vi "ShooterTest.vi"(0 "Stop Button":bool, 7 "Shooter/ArmGripper (T/F)":bool, 9 "Shoot/Load":dbl(slide)=1500.0 scale=500.0..2500.0, 10 "pitch":dbl(slide)=850.0 scale=500.0..2500.0) -> (1 "Correct Key?":bool, 2 "Battery (Volts)":dbl format="%.1f")   [LabVIEW 2019]
uses:
  <vilib>/ReMiSYS/ReMiSYS_myRIO-mini/SubVI/SYS/servoPort.ctl
panel:
  out "error out":errorcluster
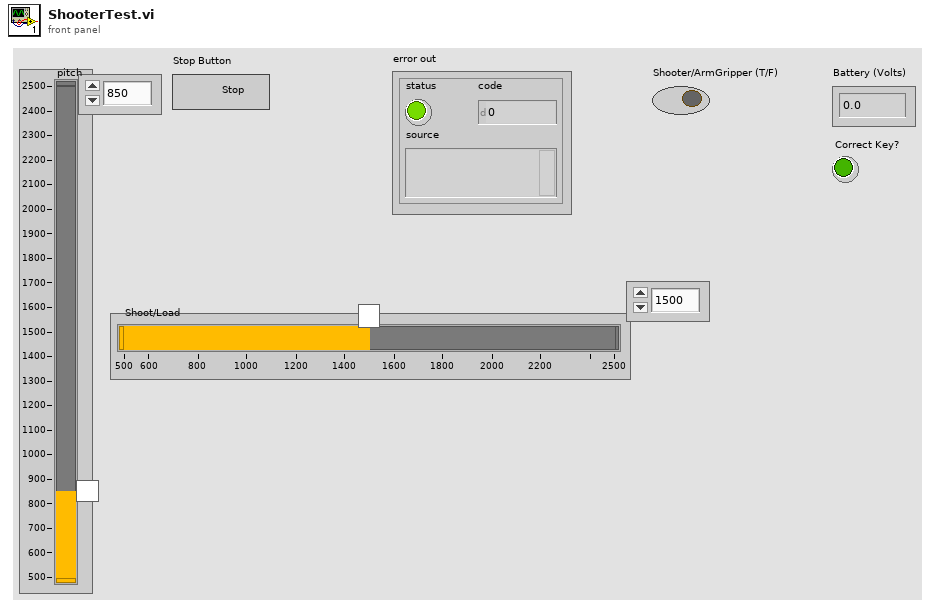
[diagram p1: front panel]
types:
  T1 = typedef "IMAQ Image.ctl" = refnum<image>
  T2 = typedef "IMAQ GM Match Report.ctl" = cluster{"Position":cluster{"x":sgl, "y":sgl}, "Angle":sgl, "Scale":sgl, "Score":sgl, "Bounding Box":cluster{"x":sgl, "y":sgl}[], "Contrast Reversed":bool, "Occlusion %":sgl, "Template Target Curve Score":sgl, "Target Template Curve Score":sgl, "Correlation Score":sgl}
  T3 = cluster{"Position":cluster{"x":sgl, "y":sgl}, "Angle":sgl, "Scale":sgl, "Score":sgl, "Bounding Box":cluster{"x":sgl, "y":sgl}[]}[]
  T4 = typedef "miniRef.ctl" = cluster{"Custom FPGA Reference":refnum<k20>, "error out":errorcluster}
  T5 = typedef "servoPort.ctl" = enum16{"S1", "S2", "S3", "S4", "S5", "S6", "S7", "S8", "S9"}
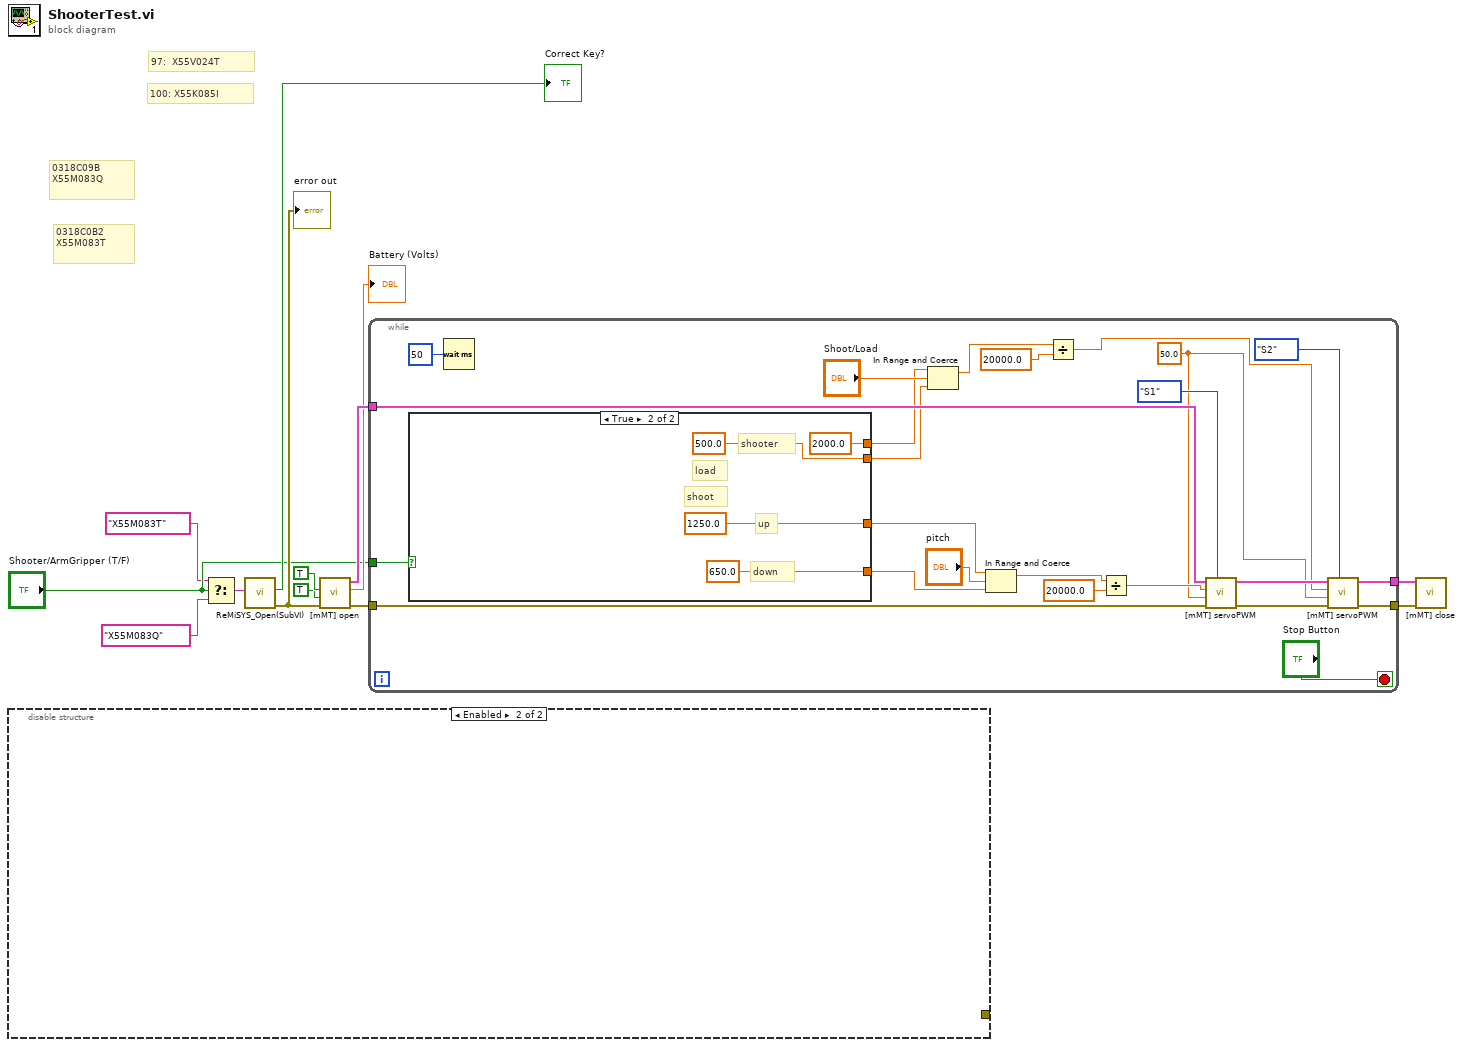
[diagram p0: block diagram]
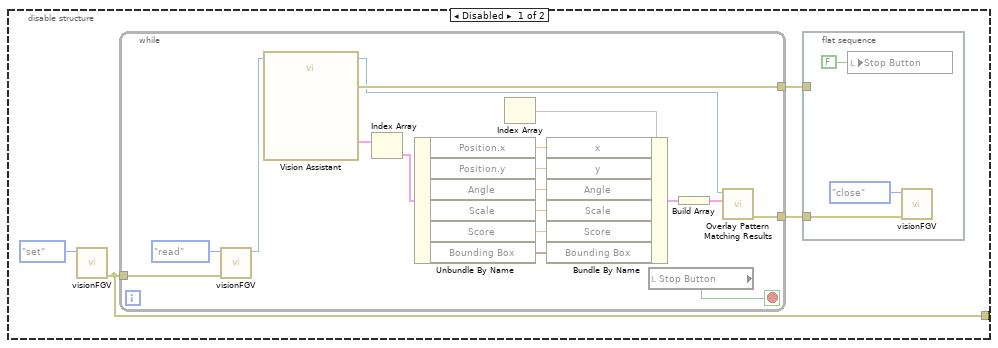
[diagram p2: hidden frame]
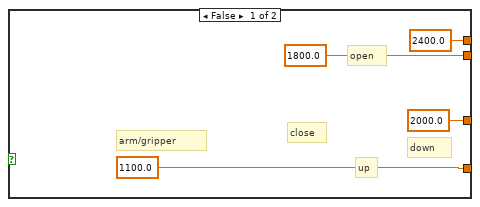
[diagram p3: hidden frame]
diagram:
  # "0318C0B2\nX55M083T"
  # "0318C09B\nX55M083Q"
  # "100: X55K085I"
  # "97:  X55V024T"
  n1 = disable-structure shown="Enabled" {
    disable-tunnel: [w16 _] -> _
    frame Disabled {
      n2 = call "visionFGV.vi"("Function"=enum16{"set", "read", "close"}."set") -> ("error out"=w16:errorcluster)  [unwired: 9 in, 1 out]
      n3 = while {
        tunnel: w16 -> [w38]
        tunnel: [w35] -> w15
        tunnel: [w21] -> w14
        stop <- w36 stop-if-true
        n4 = call "visionFGV.vi"("Error In"=w38, "Function"=enum16{"set", "read", "close"}."read") -> ("Image Out fgv"=w37:T1)  [unwired: 8 in, 1 out]
        n5 = call "Vision Assistant"("Image In"=w37) -> ("Image Out"=w34:T1, "Matches (Pattern Matching 1)"=w31:T2[], "error out"=w35:errorcluster)  [unwired: 24 in]
        n6 = Index Array(array=w31) -> (element=w30:T2)  [unwired: 1 in]
        n7 = Unbundle By Name(w30) -> ("Position.x"=w29:sgl, "Position.y"=w28:sgl, "Angle"=w27:sgl, "Scale"=w26:sgl, "Score"=w25:sgl, "Bounding Box"=w24:cluster{"x":sgl, "y":sgl}[])
        n8 = Index Array() -> (array=w33:T3, element=w32)  [unwired: 1 in]
        n9 = Bundle By Name(cluster=w32, "x"=w29, "y"=w28, "Angle"=w27, "Scale"=w26, "Score"=w25, "Bounding Box"=w24) -> (w23:cluster{})
        n10 = local read "Stop Button"() -> (w36:bool)
        n11 = Build Array(w23) -> (w22:cluster{}[])
        n12 = call "Overlay Pattern Matching Results.vi"("Matches"=w22, "Image"=w34) -> ("error out"=w21:errorcluster)  [unwired: 8 in, 1 out]
      }
      n13 = flat-sequence {
        tunnel: w15 -> [_]
        tunnel: w14 -> [w18]
        frame #0 {
          n14 = local write "Stop Button"(FALSE ("Stop Button")) -> ()
          n15 = call "visionFGV.vi"("Error In"=w18, "Function"=enum16{"set", "read", "close"}."close") -> ()  [unwired: 8 in, 2 out]
        }
      }
    }
    frame Enabled {
    }
  }
  n16 = Select(t="X55M083T" ("ReMiSYS Key"), s="Shooter/ArmGripper (T/F)", f="X55M083Q" ("ReMiSYS Key")) -> (s? t:f=w1:string)
  n17 = call <vilib>:"ReMiSYS_Open(SubVI).vi"("ReMiSYS Key"=w1) -> ("error out"=w13:errorcluster, "Correct Key?"=→"Correct Key?":bool)  [unwired: 9 in]
  "error out" <- w13
  n18 = call <vilib>:"[mMT] open.vi"("error in"=w13, "Servo8,9"=TRUE, "Servo6,7"=TRUE) -> ("error out"=w12:errorcluster, "Battery (Volts)"=→"Battery (Volts)":dbl, "miniOut"=w11:T4)  [unwired: 6 in]
  n19 = while {
    tunnel: w12 -> [w63]
    tunnel: w11 -> [w60]
    tunnel: [w46] -> w6
    tunnel: [w45] -> w5
    tunnel: "Shooter/ArmGripper (T/F)" -> [w40]
    stop <- "Stop Button" stop-if-true
    w48 = 50.0 ("Frequency")
    n20 = case shown="True" w40 {
      tunnel: [1100.0 ("lower limit") 650.0 ("lower limit")] -> w44
      tunnel: [2000.0 ("upper limit") 1250.0 ("upper limit")] -> w43
      tunnel: [1800.0 ("lower limit") 500.0 ("lower limit")] -> w42
      tunnel: [2400.0 ("upper limit") 2000.0 ("upper limit")] -> w41
      frame False {
        # "close"
        # "open"
        # "down"
        # "up"
        # "arm/gripper"
      }
      frame True {
        # "shooter"
        # "down"
        # "up"
        # "shoot"
        # "load"
      }
    }
    n21 = Wait (ms)(milliseconds to wait=u32 50) -> ()  [unwired: 1 out]
    n22 = In Range and Coerce(upper limit=w41, x="Shoot/Load", lower limit=w42) -> (coerced(x)=w54:dbl)  [unwired: 1 out]
    n23 = In Range and Coerce(upper limit=w43, x="pitch", lower limit=w44) -> (coerced(x)=w58:dbl)  [unwired: 1 out]
    n24 = Divide(x=w54, y=20000.0) -> (x/y=w47:dbl)
    n25 = Divide(x=w58, y=20000.0) -> (x/y=w56:dbl)
    n26 = call <vilib>:"[mMT] servoPWM.vi"("servoPort"=servoPort."S1", "error in (no error)"=w63, "Frequency"=w48, "DutyCycle"=w56, "miniOut in"=w60) -> ("error out"=w50:errorcluster, "miniOut out"=w49:T4)  [unwired: 5 in]
    n27 = call <vilib>:"[mMT] servoPWM.vi"("servoPort"=servoPort."S2", "error in (no error)"=w50, "Frequency"=w48, "DutyCycle"=w47, "miniOut in"=w49) -> ("error out"=w46:errorcluster, "miniOut out"=w45:T4)  [unwired: 5 in]
  }
  n28 = call <vilib>:"[mMT] close.vi"("error in (no error)"=w6, "miniOut in"=w5) -> ()  [unwired: 9 in, 1 out]
